vi "Identify.vi"(8 "error in (no error)":errorcluster, 11 "Test Measurement in":refnum<class "Test Measurement.lvclass">) -> (0 "error out":errorcluster, 2 "Plugin is Valid":bool, 3 "Test Measurement out":refnum<class "Test Measurement.lvclass">)   [LabVIEW 2016, in "Test Measurement.lvclass"]
uses:
  Test Measurement.lvclass
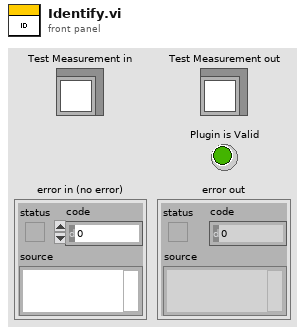
[diagram p1: front panel]
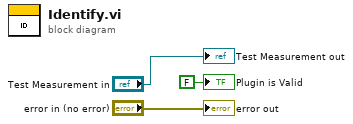
[diagram p0: block diagram]
diagram:
  "error out" <- "error in (no error)"
  "Test Measurement out" <- "Test Measurement in"
  "Plugin is Valid" <- FALSE ("Plugin is Valid")
